vi "normalizeValue.vi"(8 "error in":errorcluster caption="에러 입력", 9 "최대값":dbl=32767.0, 10 "경계값":dbl=7000.0, 11 "입력":dbl) -> (0 "error out":errorcluster caption="에러 출력", 3 "출력":dbl)   [LabVIEW 2018]
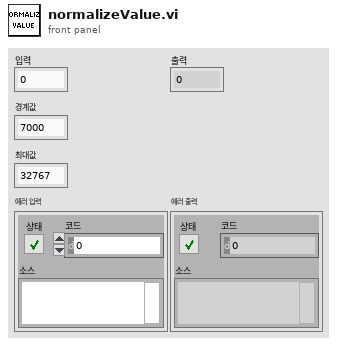
[diagram p1: front panel]
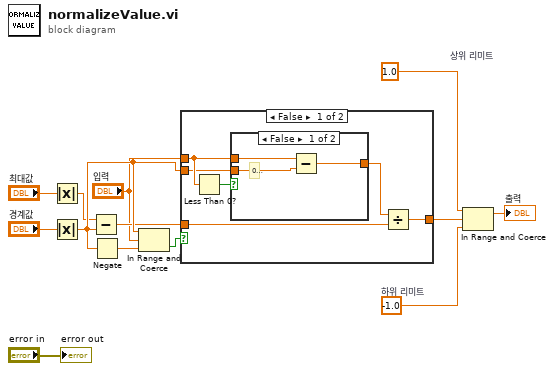
[diagram p0: block diagram]
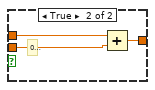
[diagram p2: hidden frame]
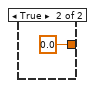
[diagram p3: hidden frame]
diagram:
  w2 = -1.0  # 하위 리미트
  w3 = 1.0  # 상위 리미트
  n1 = Absolute Value(x="최대값") -> (abs(x)=w11:dbl)
  n2 = Absolute Value(x="경계값") -> (abs(x)=w13:dbl)
  n3 = Subtract(x=w11, y=w13) -> (x-y=w12:dbl)
  n4 = Negate(x=w13) -> (-x=w6:dbl)
  n5 = In Range and Coerce(upper limit=w13, x="입력", lower limit=w6) -> (In Range?=w7:bool)  [unwired: 1 out]
  n6 = case shown="False" w7 {
    tunnel: [w14 0.0] -> w5
    tunnel: "입력" -> [w18 _]
    tunnel: w12 -> [w16 _]
    tunnel: w13 -> [w17 _]
    frame False {
      n7 = Less Than 0?(x=w18) -> (x < 0?=w19:bool)
      n8 = case shown="False" w19 {
        tunnel: w18 -> [w22 w25]
        tunnel: w17 -> [w21 w24]
        tunnel: [w20 w23] -> w15
        frame False {
          # "0이상"
          n9 = Subtract(x=w22, y=w21) -> (x-y=w20:dbl)
        }
        frame True {
          # "0보다 작음"
          n10 = Add(x=w25, y=w24) -> (x+y=w23:dbl)
        }
      }
      n11 = Divide(x=w15, y=w16) -> (x/y=w14:dbl)
    }
    frame True {
    }
  }
  n12 = In Range and Coerce(upper limit=w3, x=w5, lower limit=w2) -> (coerced(x)=→"출력":dbl)  [unwired: 1 out]
  "error out" <- "error in"
